vi "tm486_dataextraction.vi"() -> ()   [LabVIEW 2019]
panel:
  in  "r2 sy":i32=512
  in  "r2 sx":i32=512
  in  "r2 ox":i32=1024
  in  "r2 oy":i32=512
  in  "r1 sy":i32=512
  in  "r1 sx":i32=512
  in  "r1 ox":i32
  in  "r1 oy":i32=1024
  out "Timestamp":dbl
  out "DCAM Version":string
  out "Library Version":string
  out "Image":u16[][](graph)
  out "Frames Per Second":dbl
  in  "Quit":bool
  out "Error Out":errorcluster {"code" format="%.0x"}
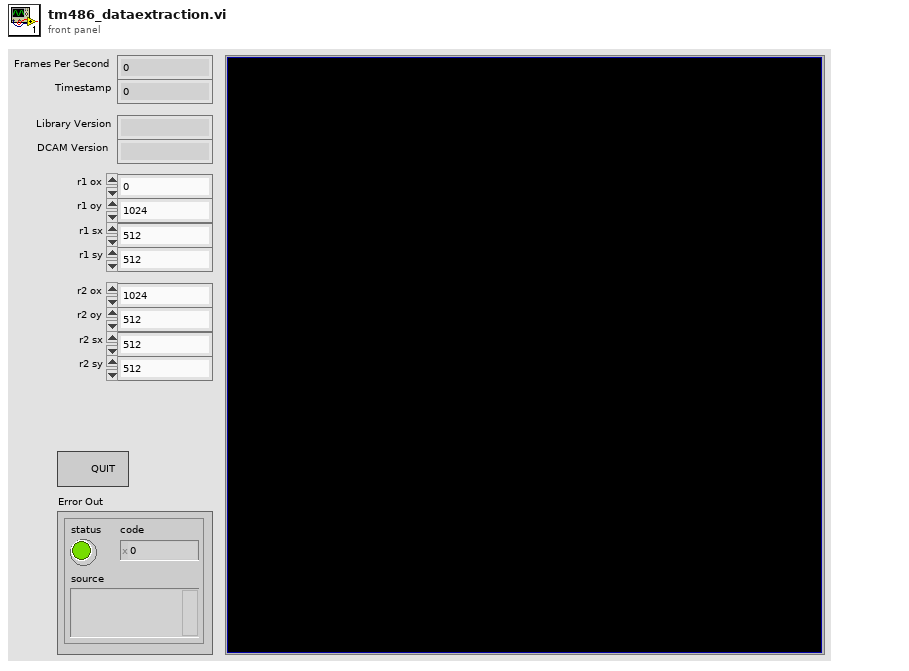
[diagram p1: front panel]
types:
  T1 = cluster{"Capture Library":string, "DCAM-API":string}
  T2 = cluster{"r1 ox":i32, "r1 oy":i32, "r1 sx":i32, "r1 sy":i32}
  T3 = cluster{"r2 ox":i32, "r2 oy":i32, "r2 sx":i32, "r2 sy":i32}
  T4 = cluster{"r2 ox":i32, "r2 oy":i32, "r2 sx":i32, "r2 sy":i32}[]
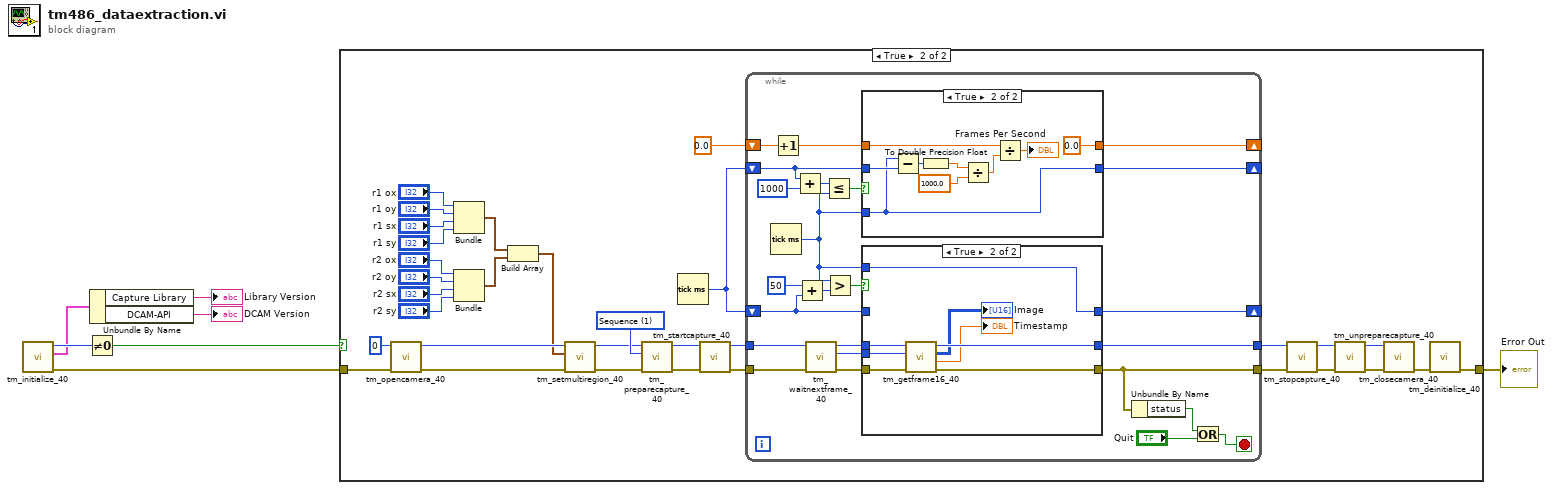
[diagram p0: block diagram]
diagram:
  n1 = call <userlib>:"tm_initialize_40.vi"() -> ("error out"=w4:errorcluster, "Version Info"=w3:T1, "Number Of Cameras"=w5:u32)  [unwired: 8 in, 1 out]
  n2 = Not Equal To 0?(x=w5) -> (x != 0?=w7:bool)
  n3 = Unbundle By Name(w3) -> ("Capture Library"=→"Library Version":string, "DCAM-API"=→"DCAM Version":string)
  n4 = case shown="True" w7 {
    tunnel: w4 -> [w8 w40]
    tunnel: [w8 w37] -> w6
    frame False {
    }
    frame True {
      w28 = 1 items=["Snap", "Sequence"] ("Capture mode")
      n5 = call <userlib>:"tm_opencamera_40.vi"("error in (no error)"=w40, "Camera Index"=u32 0) -> ("error out"=w16:errorcluster, "Handle out"=w18:u32)  [unwired: 7 in, 1 out]
      n6 = Bundle("r1 ox"="r1 ox", "r1 oy"="r1 oy", "r1 sx"="r1 sx", "r1 sy"="r1 sy") -> (w21:T2)  [unwired: 1 in]
      n7 = Bundle("r2 ox"="r2 ox", "r2 oy"="r2 oy", "r2 sx"="r2 sx", "r2 sy"="r2 sy") -> (w11:T3)  [unwired: 1 in]
      n8 = Build Array(w21, w11) -> (w17:T4)
      n9 = call <userlib>:"tm_setmultiregion_40.vi"("error in (no error)"=w16, "Sub Regions"=w17, "Handle in"=w18) -> ("error out"=w14:errorcluster, "Handle out"=w15:u32)  [unwired: 7 in]
      n10 = call <userlib>:"tm_preparecapture_40.vi"("error in (no error)"=w14, "Capture mode"=w28, "Handle in"=w15) -> ("error out"=w26:errorcluster, "Handle out"=w27:u32)  [unwired: 5 in, 2 out]
      n11 = Tick Count (ms)() -> (millisecond timer value=w24:u32)
      n12 = call <userlib>:"tm_startcapture_40.vi"("error in (no error)"=w26, "Handle in"=w27) -> ("error out"=w29:errorcluster, "Handle out"=w30:u32)  [unwired: 8 in]
      n13 = while {
        tunnel: [w43] -> w33
        tunnel: [w44] -> w34
        tunnel: w30 -> [w61]
        tunnel: w29 -> [w62]
        shift-right: [w59] -> _
        shift-left: w24 -> [w56]
        shift-right: [w60] -> _
        shift-left: 0.0 -> [w53]
        shift-right: [w42] -> _
        shift-left: w24 -> [w45]
        stop <- w41 stop-if-true
        n14 = Tick Count (ms)() -> (millisecond timer value=w46:u32)
        n15 = Increment(x=w53) -> (x+1=w54:dbl)
        n16 = Add(x=w56, y=u32 1000) -> (x+y=w58:u32)
        n17 = Add(x=u32 50, y=w45) -> (x+y=w48:u32)
        n18 = call <userlib>:"tm_waitnextframe_40.vi"("error in (no error)"=w62, "Handle in"=w61) -> ("error out"=w51:errorcluster, "Frame Index"=w50:i32, "Handle out"=w52:u32)  [unwired: 6 in, 1 out]
        n19 = Less Or Equal?(x=w58, y=w46) -> (x <= y?=w55:bool)
        n20 = Greater?(x=w46, y=w48) -> (0:w47:bool)
        n21 = case shown="True" w55 {
          tunnel: w56 -> [w77 w80]
          tunnel: [w77 w78] -> w59
          tunnel: w54 -> [w76 w84]
          tunnel: w46 -> [_ w78]
          tunnel: [w76 0.0] -> w60
          frame False {
          }
          frame True {
            n22 = Subtract(x=w78, y=w80) -> (x-y=w79:u32)
            n23 = To Double Precision Float(number=w79) -> (double precision float=w86:dbl)
            n24 = Divide(x=w86, y=1000.0) -> (x/y=w83:dbl)
            n25 = Divide(x=w84, y=w83) -> (x/y=→"Frames Per Second":dbl)
          }
        }
        n26 = case shown="True" w47 {
          tunnel: w52 -> [w67 w75]
          tunnel: w51 -> [w66 w74]
          tunnel: w50 -> [_ w68]
          tunnel: w45 -> [w65 _]
          tunnel: w46 -> [_ w73]
          tunnel: [w67 w71] -> w43
          tunnel: [w66 w72] -> w44
          tunnel: [w65 w73] -> w42
          frame False {
          }
          frame True {
            n27 = call <userlib>:"tm_getframe16_40.vi"("error in (no error)"=w74, "Frame Index"=w68, "Handle in"=w75) -> ("error out"=w72:errorcluster, "Timestamp"=→"Timestamp":dbl, "Data"=→"Image":u16[][], "Handle out"=w71:u32)  [unwired: 5 in]
          }
        }
        n28 = Unbundle By Name(w44) -> ("status"=w64:bool)
        n29 = Or(x=w64, y="Quit") -> (x .or. y?=w41:bool)
      }
      n30 = call <userlib>:"tm_stopcapture_40.vi"("error in (no error)"=w34, "Handle in"=w33) -> ("error out"=w31:errorcluster, "Handle out"=w32:u32)  [unwired: 8 in]
      n31 = call <userlib>:"tm_unpreparecapture_40.vi"("error in (no error)"=w31, "Handle in"=w32) -> ("error out"=w36:errorcluster, "Handle out"=w35:u32)  [unwired: 8 in]
      n32 = call <userlib>:"tm_closecamera_40.vi"("error in (no error)"=w36, "Handle in"=w35) -> ("error out"=w38:errorcluster)  [unwired: 9 in]
      n33 = call <userlib>:"tm_deinitialize_40.vi"("error in (no error)"=w38) -> ("error out"=w37:errorcluster)  [unwired: 10 in]
    }
  }
  "Error Out" <- w6
